vi "Close.vi"(8 "error in (no error)":errorcluster, 11 "TXT in":refnum<class "TXT.lvclass">) -> (0 "error out":errorcluster, 3 "TXT out":refnum<class "TXT.lvclass">)   [LabVIEW 2014, in "TXT.lvclass"]
uses:
  TXT.lvclass
  TXT.lvclass/TXT.ctl
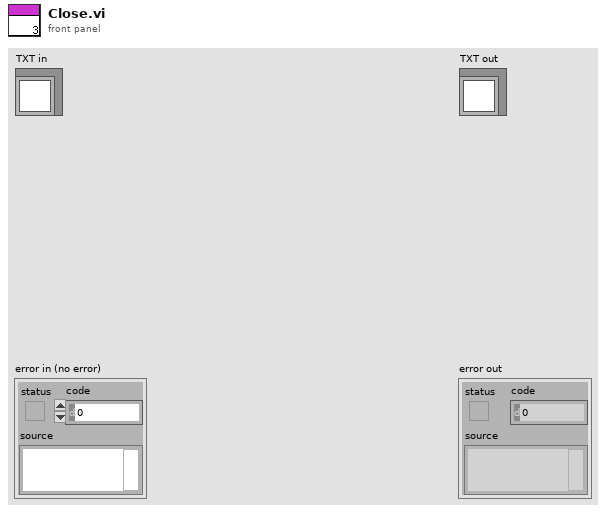
[diagram p1: front panel]
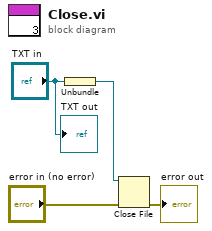
[diagram p0: block diagram]
diagram:
  n1 = Unbundle("TXT in") -> (w4:refnum<file>)
  n2 = Close File(refnum=w4, error in="error in (no error)") -> (error out=→"error out":errorcluster)  [unwired: 1 out]
  "TXT out" <- "TXT in"
